vi "Mono.step.vi"(0 "DyeLaser":T2={"Scan.Start (cm-1)"=15000.0, "Scan.Stop (cm-1)"=15050.0, "Scan.step (cm-1)"=0.2, "dye laser port"="", "Laser"=enum."Syrah", "NSteps"=251, "CurrentStep"=75, "Current.cm-1"=15015.0} {"Current.cm-1" format="%.2f"}, 5 "Mono":T1) -> (4 "DyeLaser out":T2={"Scan.Start (cm-1)"=15000.0, "Scan.Stop (cm-1)"=15050.0, "Scan.step (cm-1)"=0.2, "dye laser port"="", "Laser"=enum."Syrah", "NSteps"=251, "CurrentStep"=75, "Current.cm-1"=15015.0} {"Current.cm-1" format="%.2f"}, 6 "Mono.out":T1)   [LabVIEW 2022 SP3]
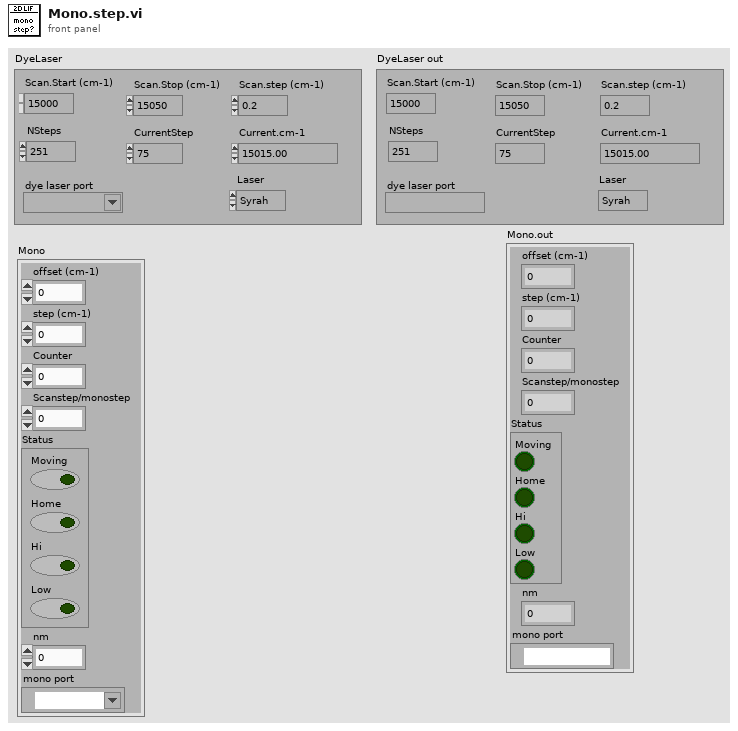
[diagram p1: front panel]
types:
  T1 = cluster{"offset (cm-1)":dbl, "step (cm-1)":dbl, "Counter":dbl, "Scanstep/monostep":i32, "Status":cluster{"Moving":bool, "Home":bool, "Hi":bool, "Low":bool}, "nm":dbl, "mono port":refnum<visa-resource-name>}
  T2 = cluster{"Scan.Start (cm-1)":dbl, "Scan.Stop (cm-1)":dbl, "Scan.step (cm-1)":dbl, "dye laser port":refnum<visa-resource-name>, "Laser":enum16{"Syrah", "Hyperdye"}, "NSteps":i32, "CurrentStep":i32, "Current.cm-1":dbl}
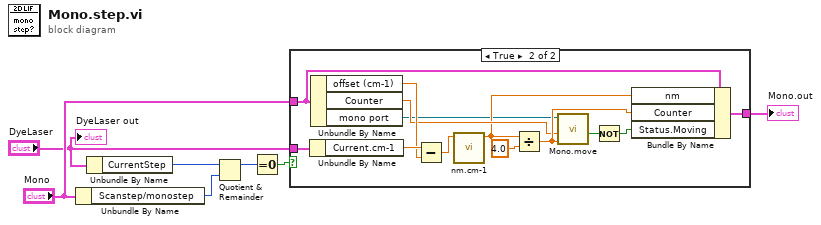
[diagram p0: block diagram]
diagram:
  n1 = Unbundle By Name("Mono") -> ("Scanstep/monostep"=w7:i32)
  n2 = Unbundle By Name("DyeLaser") -> ("CurrentStep"=w6:i32)
  n3 = Quotient & Remainder(x=w6, y=w7) -> (x-y*floor(x/y)=w3:i32)  [unwired: 1 out]
  n4 = Equal To 0?(x=w3) -> (x = 0?=w5:bool)
  n5 = case shown="True" w5 {
    tunnel: "Mono" -> [w8 w11]
    tunnel: "DyeLaser" -> [_ w18]
    tunnel: [w8 w17] -> w1
    frame False {
    }
    frame True {
      n6 = Unbundle By Name(w18) -> ("Current.cm-1"=w20:dbl)
      n7 = Unbundle By Name(w11) -> ("offset (cm-1)"=w19:dbl, "Counter"=w15:dbl, "mono port"=w12:refnum<visa-resource-name>)
      n8 = Subtract(x=w20, y=w19) -> (x-y=w14:dbl)
      n9 = call "nm.cm-1.vi"("nm or cm-1 in"=w14) -> ("cm-1 or nm  out"=w13:dbl)  [unwired: 10 in]
      n10 = Divide(x=w13, y=4.0) -> (x/y=w16:dbl)
      n11 = call "Mono.move.vi"("Target position"=w16, "Current position"=w15, "VISA resource name"=w12) -> ("done"=w10:bool)  [unwired: 8 in]
      n12 = Not(x=w10) -> (.not. x?=w9:bool)
      n13 = Bundle By Name(cluster=w11, "nm"=w13, "Counter"=w16, "Status.Moving"=w9) -> (w17:T1)
    }
  }
  "Mono.out" <- w1
  "DyeLaser out" <- "DyeLaser"
